vi "poly_detect_boolean_edges_falling.vi"(4 "tf input":bool) -> (1 "falling edge":bool)   [LabVIEW 2015]
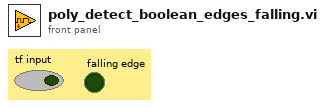
[diagram p1: front panel]
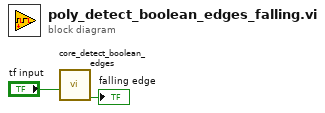
[diagram p0: block diagram]
diagram:
  n1 = call "core_detect_boolean_edges.vi"("tf input"="tf input") -> ("falling edge"=→"falling edge":bool)  [unwired: 9 in, 1 out]
